vi "Intake Testbench.vi"() -> ()   [LabVIEW 2013]
doc: "This VI imlements the framework and scheduler for your robotics program. It should not be necessary to modify the framework. You are expected to add your code to the VIs called from Robot Main, the ones located in the Team Code within the project."
uses:
  <vilib>/Rock Robotics/WPI/Joystick/WPI_JoystickDeviceEnum.ctl
  <vilib>/Rock Robotics/WPI/Solenoid/WPI_SolenoidChannel.ctl
  <vilib>/Rock Robotics/WPI/SafetyOutput/WPI_SafetyOutputConfigMenu.ctl
  <vilib>/Rock Robotics/SystemInterfaces/DIO/FPGA_DIORelayChannel.ctl
  <vilib>/Rock Robotics/SystemInterfaces/DIO/FPGA_DIOChannel.ctl
  <vilib>/Rock Robotics/WPI/Solenoid/WPI_SolenoidOpenDouble.vi
  <vilib>/Rock Robotics/WPI/MotorControl/WPI_MotorControlOpenCANJaguar.vi
  <vilib>/Rock Robotics/WPI/Counter/WPI_CounterDigitalInputToDigitalSource.vi
  <vilib>/Rock Robotics/WPI/Counter/WPI_CounterOpen Semi Period Mode.vi
  Auto Pickup Global.vi
panel:
  in  "Finish":bool
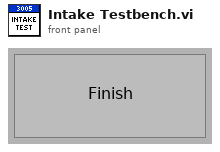
[diagram p1: front panel]
types:
  T1 = typedef "FPGA_DIOChannel.ctl" = enum8{"DIO 1", "DIO 2", "DIO 3", "DIO 4", "DIO 5", "DIO 6", "DIO 7", "DIO 8", "DIO 9", "DIO 10", "DIO 11", "DIO 12", "DIO 13", "DIO 14", "Invalid"}
  T2 = typedef "FPGA_DIORelayChannel.ctl" = enum8{"Relay 1", "Relay 2", "Relay 3", "Relay 4", "Relay 5", "Relay 6", "Relay 7", "Relay 8", "Invalid"}
  T3 = typedef "WPI_SafetyOutputConfigMenu.ctl" = enum16{"Enable", "Disable"}
  T4 = typedef "WPI_SolenoidChannel.ctl" = enum8{"Solenoid 1", "Solenoid 2", "Solenoid 3", "Solenoid 4", "Solenoid 5", "Solenoid 6", "Solenoid 7", "Solenoid 8", "Invalid"}
  T5 = typedef "WPI_JoystickDeviceEnum.ctl" = enum16{"USB 1", "USB 2", "USB 3", "USB 4", "Kinect 1", "Kinect 2"}
  T6 = typedef "WPI_CompressorDevRef.ctl" = cluster{"DevStatus":errorcluster, "DigitalInputDevRef":T7, "RelayDevRef":T9}
  T7 = typedef "WPI_DigitalInputDevRef.ctl" = cluster{"DevStatus":errorcluster, "DIO Channel":T1, "Digital Module":T8}
  T8 = typedef "FPGA_TypedefDigitalModule.ctl" = enum16{"Digital Module 1", "Digital Module 2"}
  T9 = typedef "WPI_RelayDevRef.ctl" = cluster{"DevStatus":errorcluster, "Relay Channel":T2, "Digital Module":T8, "Relay Direction":T10}
  T10 = typedef "WPI_RelayDirection.ctl" = enum16{"Both directions", "Forward only", "Reverse only"}
  T11 = typedef "WPI_JoystickDevRef.ctl" = cluster{"Device":T5}
  T12 = typedef "FPGA_CounterEncoderSourceConvertionLVSourceType.ctl" = cluster{"DevStatus":errorcluster, "AnalogTriggerMode?":bool, "DigitalMode":cluster{"Digital Module":T8, "DIO Channel":T13}, "AnalogTriggerMode":cluster{"AnalogTriggerIndex":T14, "OutputType":T15}}
  T13 = typedef "FPGA_DIODigitalSourceChannel.ctl" = enum8{"DIO 1", "DIO 2", "DIO 3", "DIO 4", "DIO 5", "DIO 6", "DIO 7", "DIO 8", "DIO 9", "DIO 10", "DIO 11", "DIO 12", "DIO 13", "DIO 14", "Disabled"}
  T14 = typedef "FPGA_AnalogTriggerIndex.ctl" = enum8{"Trig 0", "Trig 1", "Trig 2", "Trig 3", "Trig 4", "Trig 5", "Trig 6", "Trig 7", "Invalid"}
  T15 = typedef "FPGA_AnalogTriggerOutType.ctl" = enum16{"InWindow", "TriggerState", "Rising", "Falling"}
  T16 = typedef "WPI_CounterDevRef.ctl" = cluster{"DevStatus":errorcluster, "CntIndex":T17}
  T17 = typedef "FPGA_CounterCtrSystemIndex.ctl" = enum8{"Ctr 0", "Ctr 1", "Ctr 2", "Ctr 3", "Ctr 4", "Ctr 5", "Ctr 6", "Ctr 7", "Invalid"}
  T18 = typedef "WPI_JoystickButtonState.ctl" = cluster{"Button 1":bool, "Button 2":bool, "Button 3":bool, "Button 4":bool, "Button 5":bool, "Button 6":bool, "Button 7":bool, "Button 8":bool, "Button 9":bool, "Button 10":bool, "Button 11":bool, "Button 12":bool}
  T19 = typedef "WPI_MotorControlDeviceRef.ctl" = cluster{"DeviceStatus":errorcluster, "Type":enum16{"PWM", "CAN"}, "PWM":cluster{"Digital Module":T8, "PWM Channel":T20, "DeadBand":T21}, "CAN":cluster{"Device Number":u8, "Control Mode":T22, "Semaphore":T23, "Max Vout":dbl}, "Invert":bool, "TransformRef":T24, "InvTransformRef":T24}
  T20 = typedef "FPGA_DIOPWMChannel.ctl" = enum8{"PWM 1", "PWM 2", "PWM 3", "PWM 4", "PWM 5", "PWM 6", "PWM 7", "PWM 8", "PWM 9", "PWM 10", "Invalid"}
  T21 = typedef "WPI_PWMDeadband.ctl" = cluster{"Name":string, "maxPositivePwm":i32, "minPositivePwm":i32, "centerPwm":i32, "maxNegativePwm":i32, "minNegativePwm":i32, "angularRange":u16}
  T22 = typedef "WPI_CANJaguar_ControlMode.ctl" = enum8{"Percent VBus", "Current", "Speed", "Position", "Voltage"}
  T23 = typedef "Semaphore RefNum" = refnum<k1>
  T24 = typedef "WPI_PWMTransform_ConPane.ctl" = refnum<vi>
  T25 = typedef "WPI_SolenoidDevRef.ctl" = cluster{"DevStatus":errorcluster, "Solenoid Module":T26, "Forward Solenoid Channel":T4, "Reverse Solenoid Channel":T4}
  T26 = typedef "FPGA_TypedefSolenoidModule.ctl" = enum16{"Solenoid Module 1", "Solenoid Module 2"}
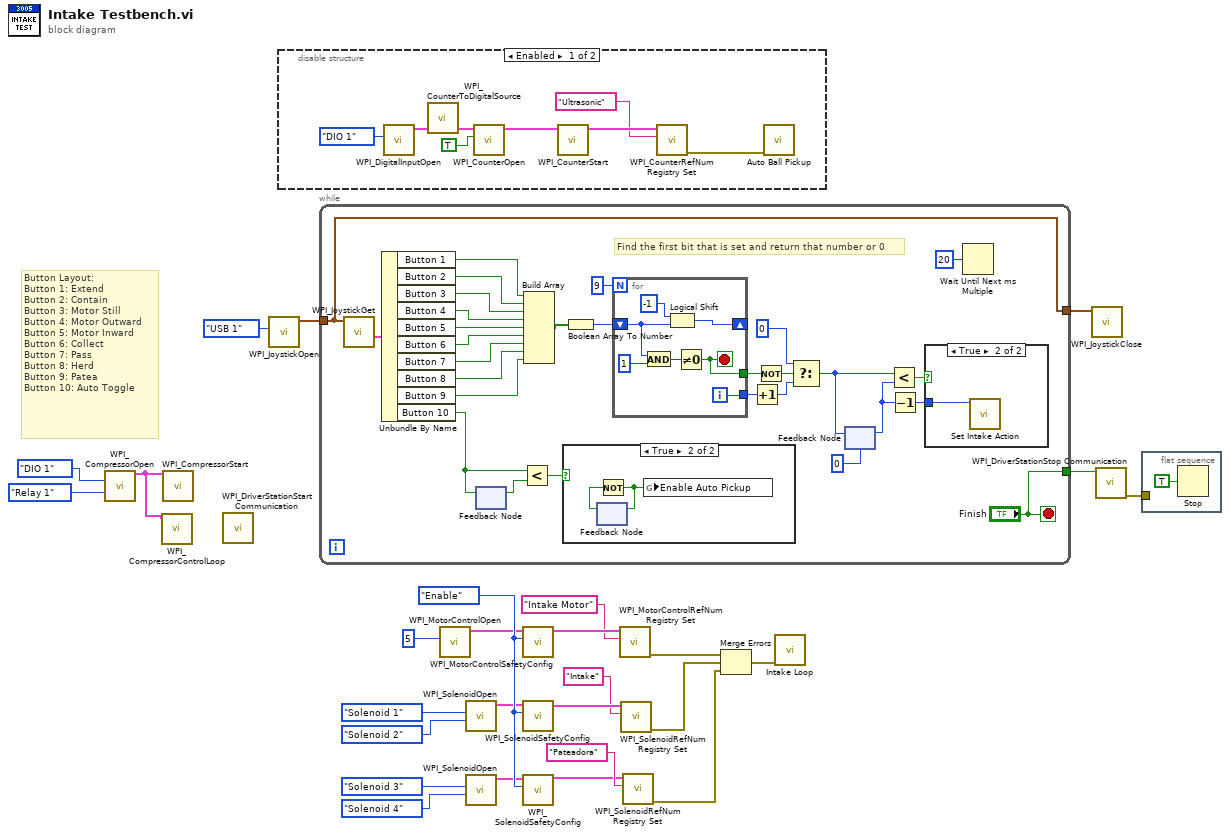
[diagram p0: block diagram]
diagram:
  w22 = WPI_SafetyOutputConfigMenu."Enable" ("mode")
  # "Button Layout:\nButton 1: Extend\nButton 2: Contain\nButton 3: Motor Still\nButton 4: Motor Outward\nButton 5: Motor Inward\nButton 6: Collect\nButton 7: Pass\nButton 8: Herd\nButton 9: Patea\nButton 10: Auto Toggle"
  n1 = call <vilib>:"WPI_CompressorOpen.vi"("Pressure Switch DIO Channel"=FPGA_DIOChannel."DIO 1", "Relay Channel"=FPGA_DIORelayChannel."Relay 1") -> ("CompressorDevRef"=w1:T6)  [unwired: 12 in, 1 out]
  n2 = call <vilib>:"WPI_CompressorControlLoop.vi"("CompressorDevRef"=w1) -> ()  [unwired: 11 in]
  n3 = call <vilib>:"WPI_CompressorStart.vi"("CompressorDevRef"=w1) -> ()  [unwired: 9 in, 2 out]
  n4 = call <vilib>:"WPI_DriverStationStart Communication.vi"() -> ()  [unwired: 1 in, 11 out]
  n5 = call <vilib>:"WPI_JoystickOpen.vi"("JoystickDevice"=WPI_JoystickDeviceEnum."USB 1") -> ("JoystickDevRef"=w27:T11)  [unwired: 10 in]
  n6 = disable-structure shown="Enabled" {
    frame Enabled {
      n7 = call <vilib>:"WPI_DigitalInputOpen.vi"("DIO Channel"=FPGA_DIOChannel."DIO 1") -> ("DigitalInputDevRef"=w34:T7)  [unwired: 2 in, 8 out]
      n8 = call-poly <vilib>:"WPI_CounterToDigitalSource.vi"("DigitalInputDevRef"=w34) -> ("Digital Source"=w32:T12)  [unwired: 6 in]
      n9 = call-poly <vilib>:"WPI_CounterOpen.vi"("High Pulse (T)"=TRUE, "Source"=w32) -> ("CounterDevRef"=w33:T16)  [unwired: 8 in, 1 out]
      n10 = call <vilib>:"WPI_CounterStart.vi"("CounterDevRef in"=w33) -> ("CounterDevRef out"=w30:T16)  [unwired: 9 in, 1 out]
      n11 = call <vilib>:"WPI_CounterRefNum Registry Set.vi"("refnum name"="Ultrasonic", "CounterDevRef"=w30) -> ("error out"=w28:errorcluster)  [unwired: 8 in, 1 out]
      n12 = call "Auto Ball Pickup.vi"("error in"=w28) -> ()  [unwired: 11 in]
    }
    frame Disabled {
    }
  }
  n13 = while {
    tunnel: ["Finish"] -> w24
    tunnel: w27 -> [w41]
    tunnel: [w41] -> w25
    stop <- "Finish" stop-if-true
    # "Find the first bit that is set and return that number or 0"
    n14 = call <vilib>:"WPI_JoystickGet.vi"("JoystickDevRef"=w41) -> ("Buttons"=w63:T18)  [unwired: 4 in, 2 out]
    n15 = Unbundle By Name(w63) -> ("Button 1"=w62:bool, "Button 2"=w61:bool, "Button 3"=w60:bool, "Button 4"=w59:bool, "Button 5"=w58:bool, "Button 6"=w57:bool, "Button 7"=w56:bool, "Button 8"=w55:bool, "Button 9"=w54:bool, "Button 10"=w38:bool)
    n16 = feedback #1() -> (w37:bool)  [unwired: 1 in]
    n17 = feedback-in #1(w38) -> ()
    n18 = Less?(x=w38, y=w37) -> (x < y?=w36:bool)
    n19 = Build Array(w62, w61, w60, w59, w58, w57, w56, w55, w54) -> (w53:bool[])
    n20 = case shown="True" w36 {
      frame False {
      }
      frame True {
        n21 = feedback #2() -> (w65:bool)  [unwired: 1 in]
        n22 = Not(x=w65) -> (.not. x?=w66:bool)
        n23 = feedback-in #2(w66) -> ()
        n24 = global write "Auto Pickup Global.vi" "Enable Auto Pickup"(w66) -> ()
      }
    }
    n25 = Boolean Array To Number(Boolean array=w53) -> (number=w52:u32)
    n26 = for {
      N: 9 -> [_]
      shift-right: [w70] -> _
      shift-left: w52 -> [w69]
      tunnel: [w72] -> w42
      tunnel: [w71] -> w51
      i -> [w72]
      stop <- w71 stop-if-true
      n27 = And(x=w69, y=u32 1) -> (x .and. y?=w73:u32)
      n28 = Logical Shift(y=i16 -1, x=w69) -> (x << y=w70:u32)
      n29 = Not Equal To 0?(x=w73) -> (x != 0?=w71:bool)
    }
    n30 = Increment(x=w42) -> (x+1=w40:i32)
    n31 = Not(x=w51) -> (.not. x?=w45:bool)
    n32 = Select(t=0, s=w45, f=w40) -> (s? t:f=w46:i32)
    n33 = feedback-in #3(w46) -> ()
    n34 = feedback #3(u32 0) -> (w44:u32)
    n35 = Less?(x=w46, y=w44) -> (x < y?=w47:bool)
    n36 = Decrement(x=w44) -> (x-1=w39:u32)
    n37 = case shown="True" w47 {
      tunnel: w39 -> [_ w67]
      frame False {
      }
      frame True {
        n38 = call "Set Intake Action.vi"("Action"=w67) -> ()  [unwired: 10 in, 1 out]
      }
    }
    n39 = Wait Until Next ms Multiple(millisecond multiple=u32 20) -> ()  [unwired: 1 out]
  }
  n40 = call-poly <vilib>:"WPI_MotorControlOpen.vi"("Device Number"=u8 5) -> ("MotorControlDeviceRef"=w19:T19)  [unwired: 9 in, 1 out]
  n41 = call-poly <vilib>:"WPI_SolenoidOpen.vi"("Reverse Solenoid Channel"=WPI_SolenoidChannel."Solenoid 2", "Forward Solenoid Channel"=WPI_SolenoidChannel."Solenoid 1") -> ("SolenoidDevRef"=w20:T25)  [unwired: 8 in, 1 out]
  n42 = call-poly <vilib>:"WPI_SolenoidOpen.vi"("Reverse Solenoid Channel"=WPI_SolenoidChannel."Solenoid 4", "Forward Solenoid Channel"=WPI_SolenoidChannel."Solenoid 3") -> ("SolenoidDevRef"=w21:T25)  [unwired: 8 in, 1 out]
  n43 = call <vilib>:"WPI_MotorControlSafetyConfig.vi"("mode"=w22, "MotorControlDevRef"=w19) -> ("MotorControlDevRef"=w14:T19)  [unwired: 8 in, 1 out]
  n44 = call <vilib>:"WPI_SolenoidSafetyConfig.vi"("mode"=w22, "SolenoidDevRef"=w20) -> ("SolenoidDevRef 2"=w13:T25)  [unwired: 8 in, 1 out]
  n45 = call <vilib>:"WPI_SolenoidSafetyConfig.vi"("mode"=w22, "SolenoidDevRef"=w21) -> ("SolenoidDevRef 2"=w9:T25)  [unwired: 8 in, 1 out]
  n46 = call <vilib>:"WPI_MotorControlRefNum Registry Set.vi"("refnum name"="Intake Motor", "MotorControlDevRef"=w14) -> ("error out"=w8:errorcluster)  [unwired: 8 in, 1 out]
  n47 = call <vilib>:"WPI_SolenoidRefNum Registry Set.vi"("refnum name"="Intake", "SolenoidDevRef"=w13) -> ("error out"=w7:errorcluster)  [unwired: 8 in, 1 out]
  n48 = call <vilib>:"WPI_SolenoidRefNum Registry Set.vi"("refnum name"="Pateadora", "SolenoidDevRef"=w9) -> ("error out"=w6:errorcluster)  [unwired: 8 in, 1 out]
  n49 = Merge Errors(w8, w7, w6) -> (w5:errorcluster)
  n50 = call "Intake Loop.vi"("error in (no error)"=w5) -> ()  [unwired: 11 in]
  n51 = call <vilib>:"WPI_JoystickClose.vi"("JoystickDevRef"=w25) -> ()  [unwired: 11 in]
  n52 = call <vilib>:"WPI_DriverStationStop Communication.vi"("StopCommunication"=w24) -> ("error out"=w23:errorcluster)  [unwired: 1 in, 9 out]
  n53 = flat-sequence {
    tunnel: w23 -> [_]
    frame #0 {
      n54 = Stop(stop? (T)=TRUE) -> ()
    }
  }
